vi "ConvertSDFto3DView.vi"(2 "SceneGraphDisp Refnum":refnum<vi>, 3 "urdf":string) -> (0 "3D Picture":refnum<vi>(3d-picture), 1 "rest of sdf":string)   [LabVIEW 2010]
uses:
  <vilib>/picture/3D Picture Control/NI_3D Picture Control.lvlib
  <vilib>/Utility/miscctls.llb/LV3DPointTypeDef.ctl
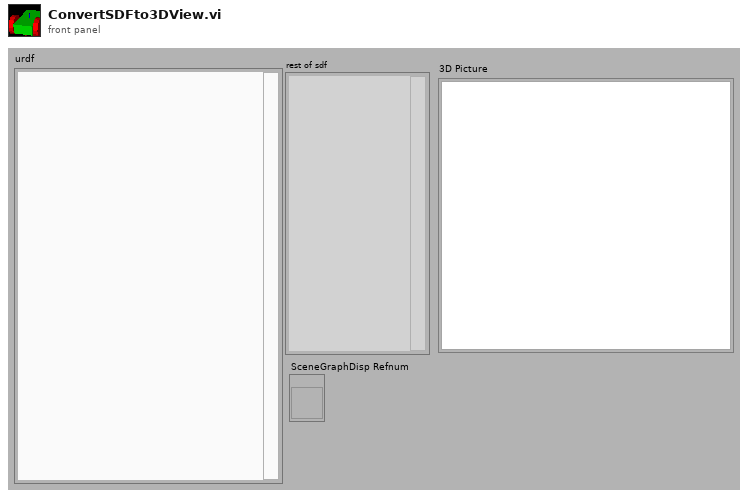
[diagram p1: front panel]
types:
  T1 = typedef "LV3DPointTypeDef.ctl" = cluster{"X":sgl, "Y":sgl, "Z":sgl}
  T2 = enum16{"None", "Spherical", "Flying", "Oriented"}
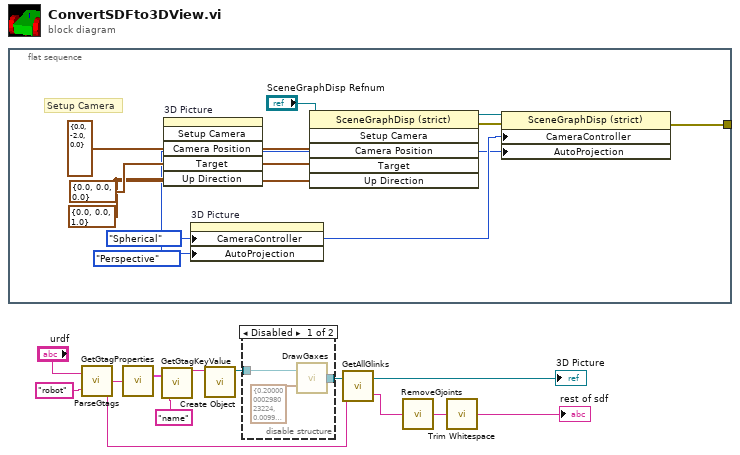
[diagram p0: block diagram]
diagram:
  n1 = flat-sequence {
    tunnel: [w14] -> _
    frame #0 {
      w21 = T1 {"X"=0.0, "Y"=-2.0, "Z"=0.0} ("Camera Position")
      w19 = T1 {"X"=0.0, "Y"=0.0, "Z"=1.0} ("Up Direction")
      w20 = T1 {"X"=0.0, "Y"=0.0, "Z"=0.0} ("Target")
      w15 = enum16{"None", "Perspective", "Orthographic"}."Perspective" ("Automatic Projection Mode")
      w16 = T2."Spherical" ("Camera Controller:Type")
      # "Setup Camera"
      n2 = invoke on="3D Picture" class="SceneGraphDisp (strict)" method="Setup Camera"("Camera Position"=w21, "Target"=w20, "Up Direction"=w19) -> ()  [unwired: 3 in, 6 out]
      n3 = property on="3D Picture" class="SceneGraphDisp (strict)"("CameraController"=w16, "AutoProjection"=w15) -> ()  [unwired: 2 in, 2 out]
      n4 = invoke on="Invoke Node" class="SceneGraphDisp (strict)" method="Setup Camera"(reference="SceneGraphDisp Refnum", "Camera Position"=w21, "Target"=w20, "Up Direction"=w19) -> (reference out=w18:refnum<vi>, error out=w17:errorcluster)  [unwired: 2 in, 4 out]
      n5 = property on="Property Node" class="SceneGraphDisp (strict)"(reference=w18, error in=w17, "CameraController"=w16, "AutoProjection"=w15) -> (error out=w14:errorcluster)  [unwired: 1 out]
    }
  }
  n6 = call "ParseGtags.vi"("tag"="robot", "urdf in"="urdf") -> ("parameters"=w6:string, "contents"=w8:string)  [unwired: 2 out]
  n7 = call "GetGtagProperties.vi"("parameters"=w6) -> ("Parameters"=w7:cluster{"key":string, "value":string}[])
  n8 = call "GetGtagKeyValue.vi"("tag"="name", "parameters"=w7) -> ("value"=w4:string)
  n9 = call <vilib>:"Create Object.vi"("Name"=w4) -> ("Scene:New Object"=w13:refnum<vi>)  [unwired: 1 in, 9 out]
  n10 = disable-structure shown="Disabled" {
    disable-tunnel: w13 -> [w25 w26]
    disable-tunnel: [w24 w26] -> w11
    frame Disabled {
      n11 = call "DrawGaxes.vi"("Shape"=cluster{"length":sgl, "width/height":sgl} {"length"=0.2, "width/height"=0.01}, "world in"=w25) -> ("world out"=w24:refnum<vi>)
    }
    frame Enabled {
    }
  }
  n12 = call "GetAllGlinks.vi"("sdf in"=w8, "Model In"=w11) -> ("remaining"=w3:string, "Model Out"=→"3D Picture":refnum<vi>)
  n13 = call "RemoveGjoints.vi"("remaining 2"=w3) -> ("remaining"=w2:string)
  n14 = call <vilib>:"Trim Whitespace.vi"("string"=w2) -> ("trimmed string"=→"rest of sdf":string)  [unwired: 1 in]
